vi "Dashboard Main.vi"() -> ()   [LabVIEW 2014]
uses:
  Robot/Auto/Autonomous Modes.ctl
  Robot/Main/Arms/Arm clapper state.ctl
  Robot/Main/Arms/Arm State.ctl
  Dashboard Tab.ctl
  <vilib>/event_ctls.llb/eventvkey.ctl
  <vilib>/vision/Image Controls.llb/IMAQ Image.ctl
  <vilib>/Rock Robotics/WPI/Dashboard/WPI_DashboardLogging Global.vi
  <vilib>/Rock Robotics/Network Tables/SD Write Number.vi
  <vilib>/Rock Robotics/Network Tables/SD Read Number.vi
  <vilib>/Rock Robotics/Network Tables/SD Write Boolean.vi
  <vilib>/Utility/config.llb/Write Key (String).vi
  <vilib>/Utility/config.llb/Write Key (I32).vi
  <vilib>/Utility/config.llb/NI_LVConfig.lvlib
  <vilib>/vision/NI_Vision_Development_Module.lvlib
panel:
  in  "Rec Mode":enum32{"Stop", "Record", "Playback"}(radio)
  in  "Vision":u16(ring) items=["Camera Off", "USB Camera SW", "USB Camera HW", "IP Camera"]
  out "fps":dbl format="%#.1g"
  out "Mbps":dbl format="%#.1g"
  out "Mbps 2":bool
  in  "TCP":refnum<k5>
  out "Camera IP":string
  out "Image Message":string="Timeout in Camera Communications"
  out "Camera Image":T1(plugin-control)
  in  "Dashboard Tab":T2(tab)
  out "Clapper Manual":bool caption="Clapper"
  out "Arm Angle Manual":bool caption="Arms"
  out "Elevator Manual":bool caption="Elevator"
  out "Arm Angle POT":dbl caption="Arm Angle"
  out "Clapper POT":dbl caption="Clapper"
  out "Left Drive Encoder":dbl caption="Left Drive"
  out "Right Drive Encoder":dbl caption="Right Drive"
  out "Elevator Encoder":dbl caption="Elevator"
  out "Version":string
  out "Arm Angle Ground":bool
  out "Arm Angle Level":bool
  out "Arm Angle Feeder":bool
  out "Arm Angle Vertical":bool
  out "Arm Angle":T3
  out "Clapper In":bool
  out "Clapper Tote":bool
  out "Clapper Bin":bool
  out "Clapper Out":bool
  out "Clapper":T4
  out "Clapper Straight":bool
  out "Motor Ramp":bool caption="Ramp"
  out "Half Drive":bool caption="Half"
  out "Mode":T5(ring)=enum."Auto Disabled"
  out "Elevator":u16
  out "Ground":bool
  out "Tote 1":bool
  out "Tote 2":bool
  out "Tote 3":bool
  out "Tote 4":bool
  out "Tote 5":bool
  out "Gyro Indicator":dbl(knob) scale=0.0..360.0
  out "Bottom LS":bool
  out "Top LS":bool
  out "Tote Detect":bool
  in  "Auto Modes":T6
  in  "DB Camera Config":bool
  in  "Camera Settings":T7={"Frame Rate"=30, "Compression"=30, "Size"=1} {"Frame Rate" scale=1.0..30.0; "Size" items=["640x480", "320x240", "160x120"]}
  in  "Test Slider":dbl(slide) scale=0.0..100.0 scale format="%#_3g"
  in  "On/Off":bool caption="Solenoid"
  in  "Test Name":u16(ring) items=["Select the test to run..."]
  in  "Test Tree":string(tree)
  in  "Motor":cluster{"Value":dbl, "Enable":bool} {"Value" scale=-1.0..1.0 scale format="%#_3g"}
  out "Progress":T8 {"Test Progress" scale=0.0..100.0}
  in  "Rev/Fwd":cluster{"Forward":bool, "Reverse":bool}
  in  "Test Ring":u16(ring) items=["Monochrome", "Color"]
  in  "Listbox":i32(listbox)
  out "Tree":string(tree)
  in  "Strafe Ramp":dbl(slide)=0.5 min=0.1 max=5.0 step=1e-06 scale=0.0..1.0
  in  "Rotate Sensitivity":dbl(slide)=1.0 min=0.0 max=1.0 step=0.05 scale=0.0..1.0
  in  "Strafe Sensitivity":dbl(slide)=1.0 min=0.0 max=1.0 step=0.05 scale=0.0..1.0
  in  "Motor Ramp":dbl(slide)=0.5 min=0.1 max=5.0 step=1e-06 scale=0.0..1.0
  in  "Joystick Curve Power":dbl=1.0 min=0.5 max=4.0 step=0.5
  in  "Elevator PIDs":bool
  in  "Strafe PIDs":bool
  in  "Arm PIDs":bool
  out "Boolean":bool
  # "POTENTIOMETERS"
  # "ENCODERS"
  # "Elevator LS"
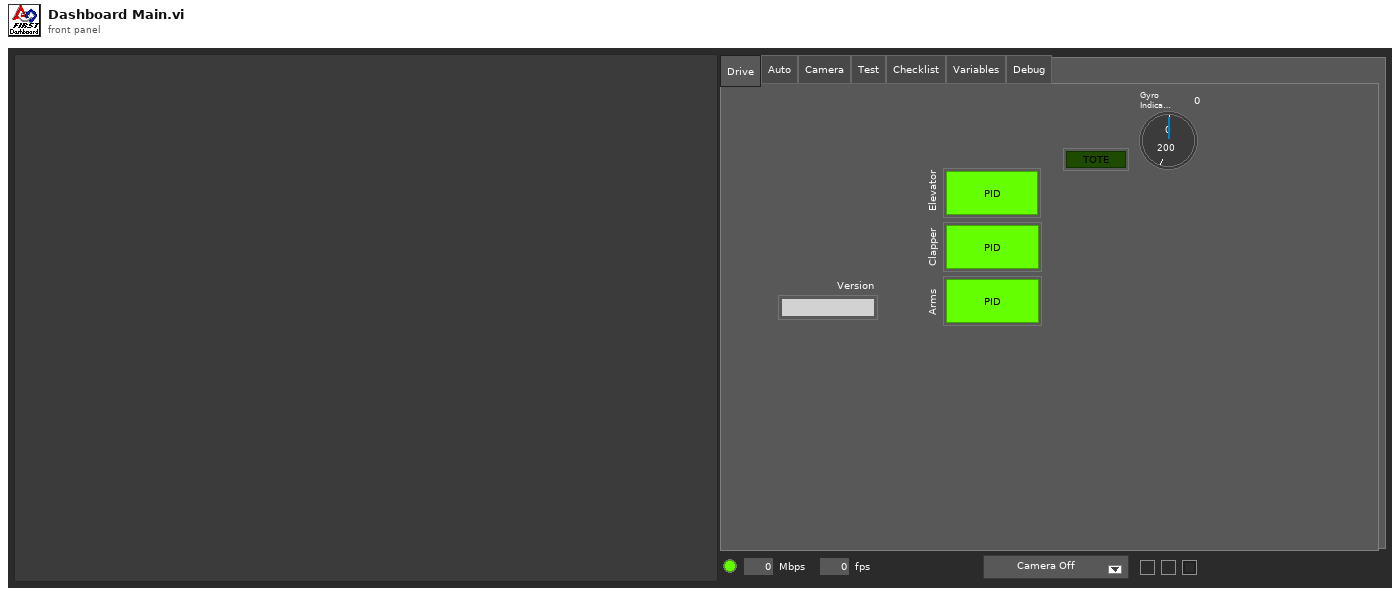
[diagram p1: front panel]
types:
  T1 = typedef "IMAQ Image.ctl" = refnum<image>
  T2 = enum32{"Drive", "Auto", "Camera", "Test", "Checklist", "Variables", "Debug"}
  T3 = typedef "Arm State.ctl" = enum16{"Ground", "Level", "Feeder", "Vertical"}
  T4 = typedef "Arm clapper state.ctl" = enum16{"In", "Tote Closed", "Bin Closed", "Straight", "Open"}
  T5 = enum8{"Tele-Op Disabled", "Tele-Op Enabled", "Auto Disabled", "Auto Enabled", "Test Disabled", "Test Enabled", "Disconnected", "No Code", "E-Stop"}
  T6 = typedef "Autonomous Modes.ctl" = enum16{"3 Tote", "Turn Left, Drive to Auto", "Turn Right, Drive to Auto", "1 Bin", "Move To Auto Zone", "Do Nothing"}
  T7 = cluster{"Frame Rate":i32, "Compression":i32, "Size":u16}
  T8 = cluster{"Test Progress":u8, "Test Progress Text":string}
  T9 = typedef "Dashboard Tab.ctl" = enum16{"Drive", "Auto", "Camera", "Test", "Checklist", "Variables", "Debug"}
  T10 = typedef "Image Type" = u32
  T11 = cluster{"Camera Image":refnum<vi>, "Dashboard Tab":refnum<vi>, "Boolean":refnum<vi>, "Vision":refnum<vi>, "Rec Mode":refnum<vi>, "Test Slider":refnum<vi>, "On/Off ":refnum<vi>, "Test Ring":refnum<vi>, "Rev/Fwd":refnum<vi>, "Test Name":refnum<vi>, "Motor":refnum<vi>, "Progress":refnum<vi>, "CheckList":refnum<vi>, "Tree":refnum<vi>, "Test Tree":refnum<vi>}
  T12 = cluster{"Error Strings":string, "Disable Counts":cluster{u16, u16}, "Rail Faults":cluster{u16, u16, u16}, "Robot IP":string, "DB Mode":u8, "Event Info":cluster{"Name":string, "Type":u8, "Number":u16, "Replay":u8}, "Camera Addr":string}
  T13 = cluster{"Storage":cluster{"Disk Free":u64, "RAM Block":u32, "RAM free":u32}, "CPU Utilization":cluster{"CPU % ISR":sgl, "CPU % Time Crit":sgl, "CPU % Timed Str":sgl, "CPU % High":sgl, "CPU % Above":sgl, "CPU % Normal":sgl, "CPU % Low":sgl}, "CAN":cluster{"% Bus Utilization":sgl, "Bus Off Cnt":u32, "TX_FIFO Full Cnt":u32, "Receive Error Cnt":u8, "Transmit Error Cnt":u8}, "HID":cluster{"HID Outputs":u32, "Rumble Low":u16, "Rumble High":u16}[]}
  T14 = cluster{"Status bits":cluster{"Test Mode":bool, "Autonomous":bool, "Enabled":bool, "Code Start":bool, "Brownout":bool, "Reserved 2":bool, "Reserved 3":bool, "E-Stop":bool}, "Code Trace":cluster{"Disabled":bool, "TeleOp":bool, "Auto":bool, "Test":bool}, "Controller Type":enum16{"unknown", "cRIO", "roboRio"}, "Code?":enum16{"unknown", "noCode", "code"}, "Battery V":dbl}
  T15 = cluster{"Control Bits":cluster{"TestMode":bool, "Autonomous":bool, "Enabled":bool, "FMS Present":bool, bool, bool, bool, "E-Stop":bool}, "Team Station ":u8, "Countdown":sgl, "Joystick Values":cluster{"Axes":dbl[], "Buttons":bool[], "POVs":i16[]}[]}
  T16 = cluster{"Axes":dbl[], "Buttons":bool[], "POVs":i16[]}[]
  T17 = cluster{"Axes":dbl[], "Buttons":bool[], "POVs":i16[]}
  T18 = typedef "NI_LVConfig.lvlib/Config Data RefNum.ctl" = refnum<k1>
  T19 = cluster{"Operation":enum16{"Update", "Clear"}, "Color Box":u32}[]
  T20 = typedef "eventvkey.ctl" = enum16{"ASCII", "Enter", "Return", "Shift", "Ctrl", "Alt", "Cmd", "Opt", "Caps", "NumLock", "Clear", "Break", "Up", "Down", "Left", "Right", "Insert", "Delete", "Home", "End", "PageUp", "PageDown", "Escape", "Help", "Pause", "ScrollLock", "F1", "F2", "F3", "F4", "F5", "F6", "F7", "F8", "F9", "F10", "F11", "F12", "F13", "F14", "F15", "F16", "F17", "F18", "F19", "F20", "F21", "F22", "F23", "F24", "Play", "VolumeUp", "VolumeDown", "Mute", "Two Byte Char"}
  T21 = cluster{"Image Size":bool, "Image Type":bool, "Pixel Value":bool, "ROI Information":bool, "Zoom Factor":bool}
  T22 = enum8{"Enabled", "Disabled", "Disabled and Grayed Out"}
  T23 = cluster{"Operation":enum16{"Update", "Clear"}, "Color Box":u32}
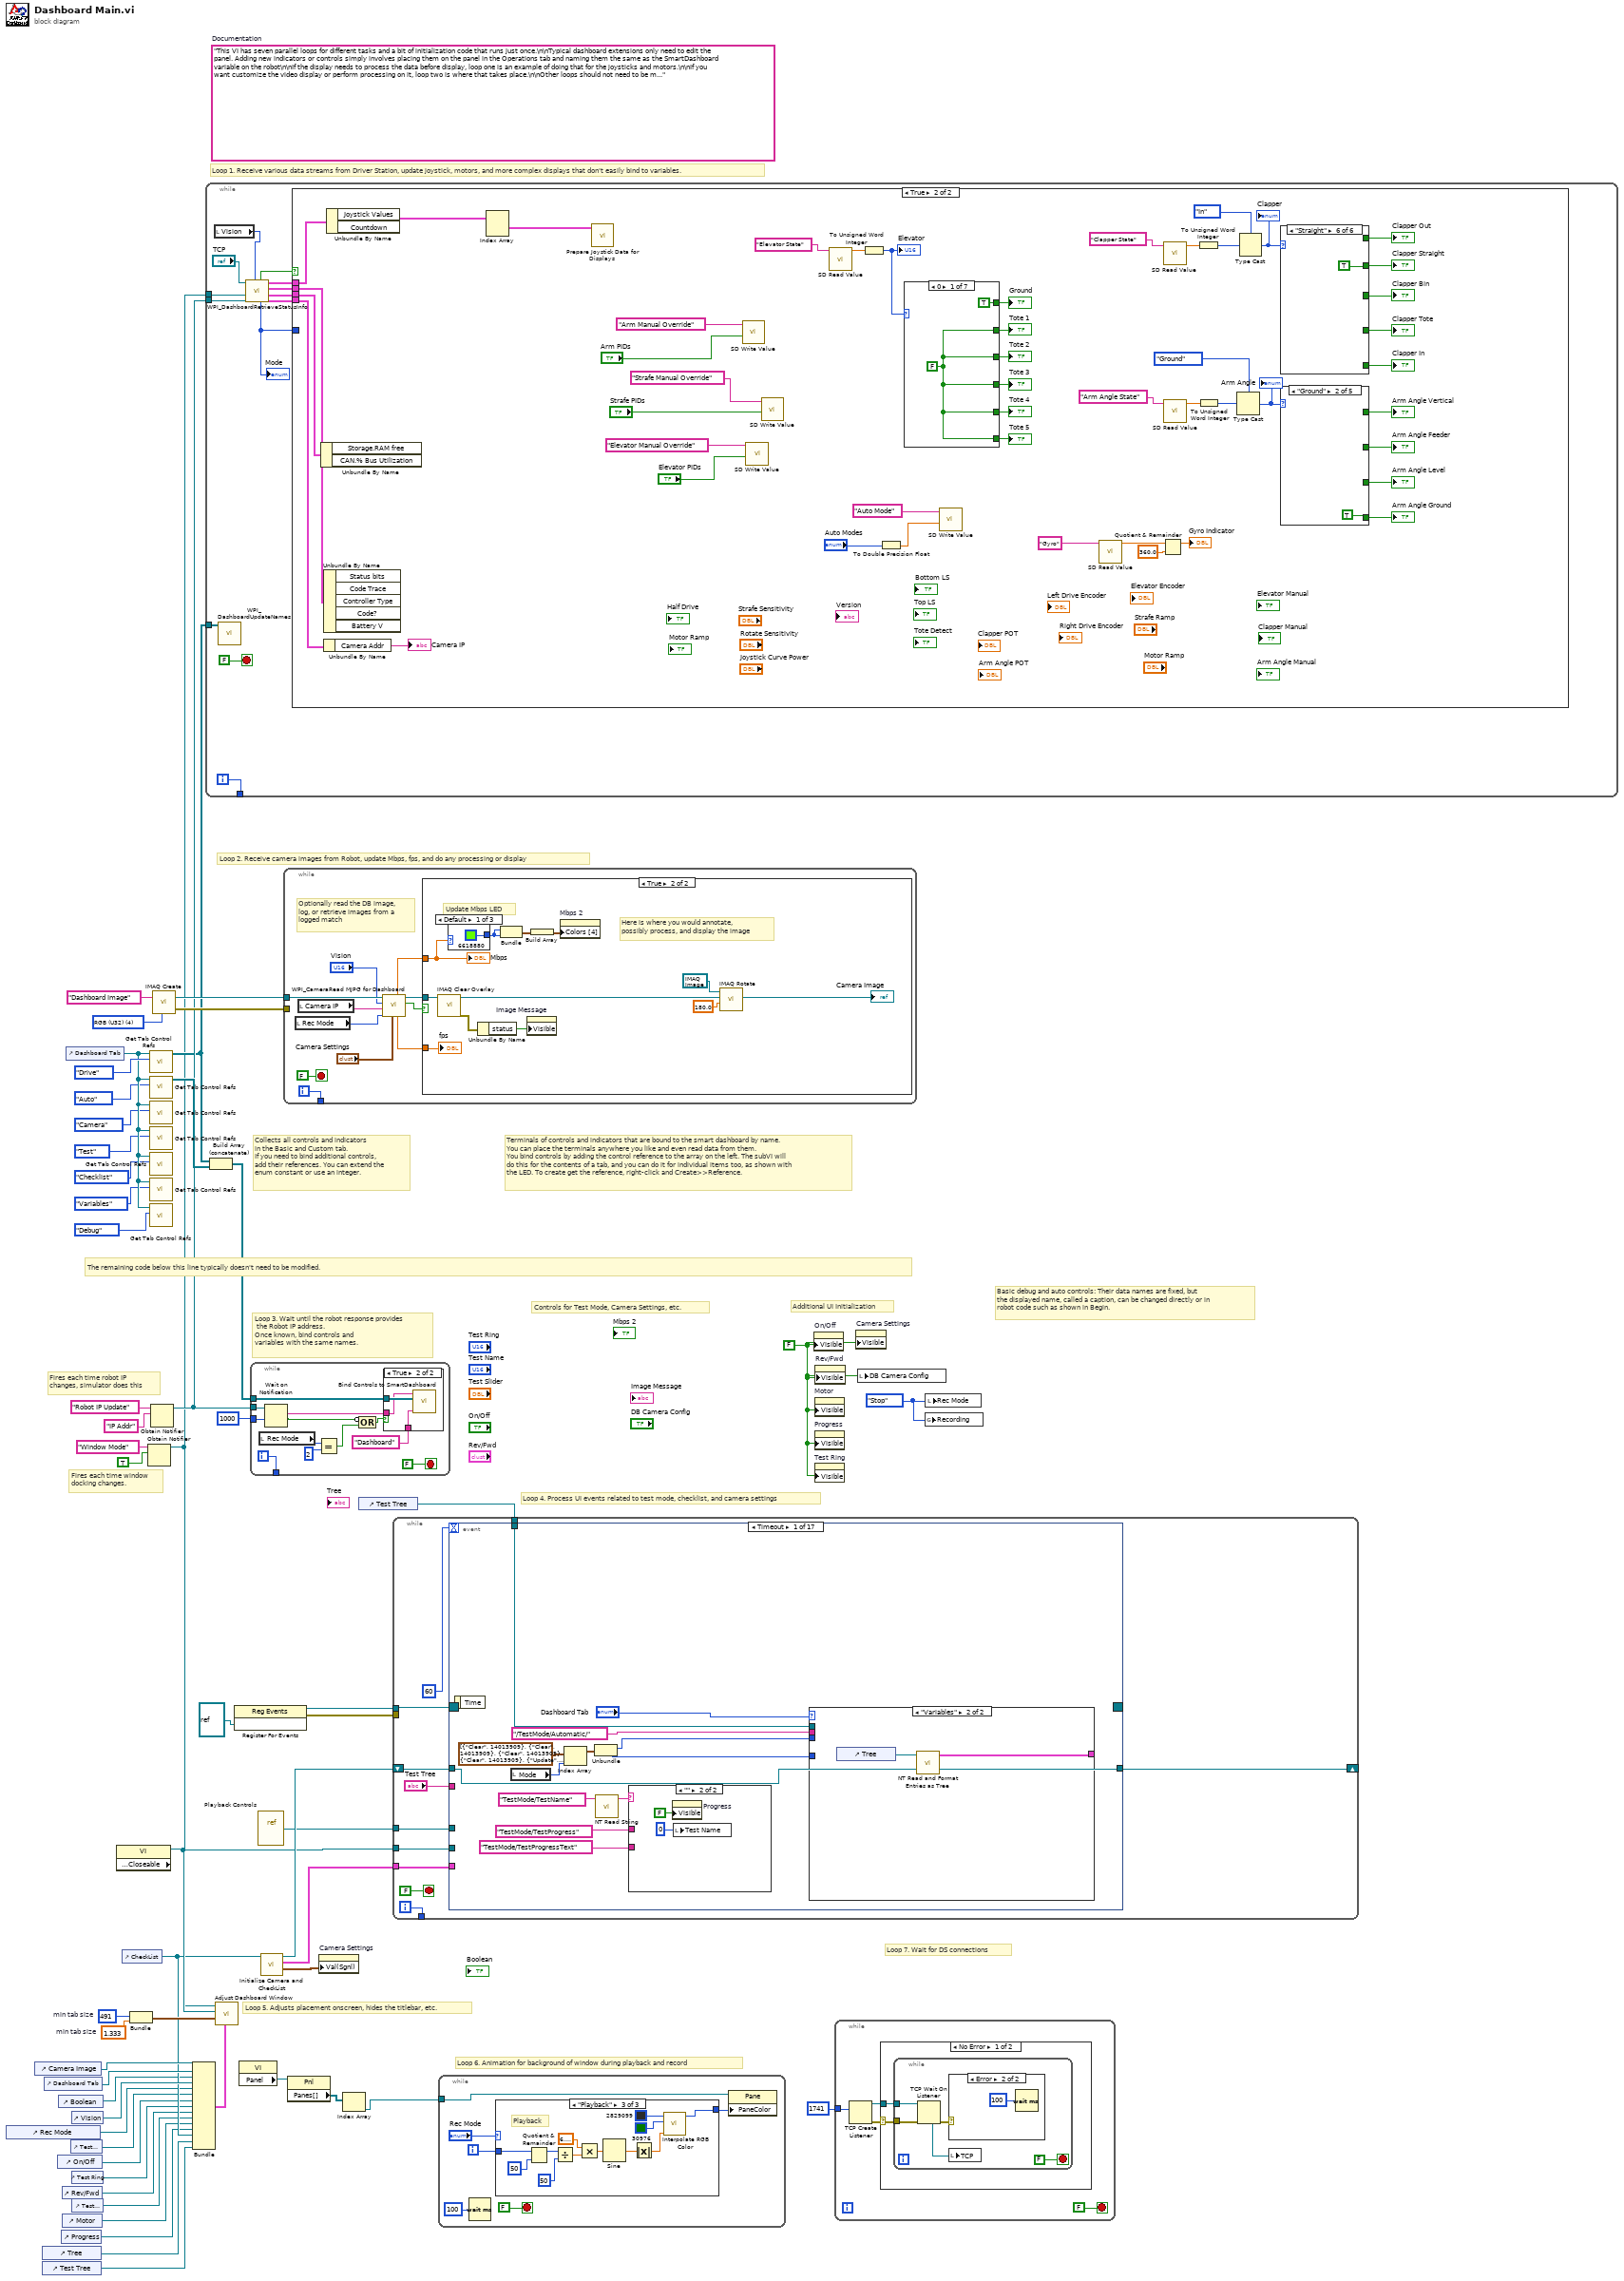
[diagram p0: block diagram]
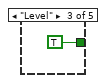
[diagram p6: hidden frame]
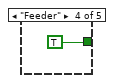
[diagram p7: hidden frame]
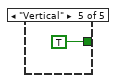
[diagram p8: hidden frame]
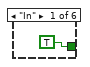
[diagram p9: hidden frame]
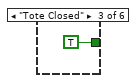
[diagram p11: hidden frame]
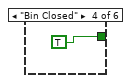
[diagram p12: hidden frame]
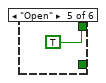
[diagram p13: hidden frame]
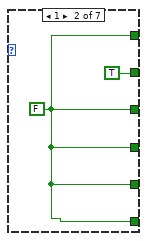
[diagram p14: hidden frame]
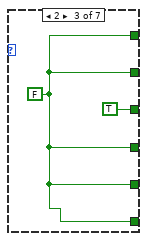
[diagram p15: hidden frame]
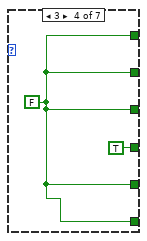
[diagram p16: hidden frame]
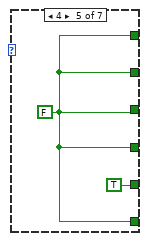
[diagram p17: hidden frame]
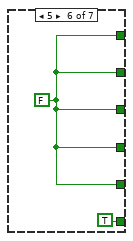
[diagram p18: hidden frame]
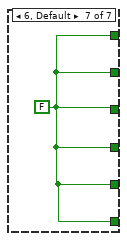
[diagram p19: hidden frame]
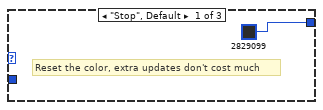
[diagram p20: hidden frame]
diagram:
  w29 = 491  # min tab size
  w28 = 1.333  # min tab size
  w36 = enum32{"Stop", "Record", "Playback"}."Stop" ("Rec Mode")
  w15 = FALSE ("Visible")
  (unwired) "This VI has seven parallel loops for different tasks and a bit of initialization code that runs just once.\n\nTypical dashboard extensions only need to edit the panel. Adding new indicators or controls simply involves placing them on the panel in the Operations tab and naming them the same as the SmartDashboard variable on the robot\n\nIf the display needs to process the data before display, loop one is an example of doing that for the joysticks and motors.\n\nIf you want customize the video display or perform processing on it, loop two is where that takes place.\n\nOther loops should not need to be modified. They are pretty standard, and document the task they perform."  # Documentation
  w56 = T10 4 items=["Grayscale (U8)", "Grayscale (I16)", "Grayscale (SGL)", "Complex (CSG)", "RGB (U32)", "HSL (U32)", "RGB (U64)"] ("Image Type")
  # "Loop 7. Wait for DS connections"
  # "Basic debug and auto controls: Their data names are fixed, but\nthe displayed name, called a caption, can be changed directly or in\nrobot code such as shown in Begin."
  # "Controls for Test Mode, Camera Settings, etc."
  # "Additional UI Initialization"
  # "Loop 6. Animation for background of window during playback and record"
  # "Fires each time robot IP\nchanges, simulator does this"
  # "Fires each time window\ndocking changes."
  # "Collects all controls and indicators\nin the Basic and Custom tab.\nIf you need to bind additional controls,\nadd their references. You can extend the\nenum constant or use an integer."
  # "The remaining code below this line typically doesn't need to be modified."
  # "Loop 4. Process UI events related to test mode, checklist, and camera settings"
  # "Terminals of controls and indicators that are bound to the smart dashboard by name.\nYou can place the terminals anywhere you like and even read data from them.\nYou bind controls by adding the control reference to the array on the left. The subVI will\ndo this for the contents of a tab, and you can do it for individual items too, as shown with\nthe LED. To create get the reference, right-click and Create>>Reference."
  # "Loop 3. Wait until the robot response provides\n the Robot IP address.\nOnce known, bind controls and\nvariables with the same names."
  # "Loop 5. Adjusts placement onscreen, hides the titlebar, etc."
  # "Loop 1. Receive various data streams from Driver Station, update joystick, motors, and more complex displays that don't easily bind to variables."
  # "Loop 2. Receive camera images from Robot, update Mbps, fps, and do any processing or display"
  n1 = control-ref of="Rec Mode"() -> (w21:refnum<vi>)
  n2 = control-ref of="Camera Image"() -> (w32:refnum<vi>)
  n3 = control-ref of="Tree"() -> (w25:refnum<vi>)
  n4 = control-ref of="Test Tree"() -> (w24:refnum<vi>)
  n5 = control-ref of="Dashboard Tab"() -> (w31:refnum<vi>)
  n6 = control-ref of="On/Off"() -> (w19:refnum<vi>)
  n7 = control-ref of="Boolean"() -> (w1:refnum<vi>)
  n8 = control-ref of="Progress"() -> (w16:refnum<vi>)
  n9 = control-ref of="Rev/Fwd"() -> (w17:refnum<vi>)
  n10 = control-ref of="Motor"() -> (w22:refnum<vi>)
  n11 = control-ref of="Dashboard Tab"() -> (w9:refnum<vi>)
  n12 = control-ref of="Test Slider"() -> (w20:refnum<vi>)
  n13 = control-ref of="Vision"() -> (w30:refnum<vi>)
  n14 = control-ref of="Test Ring"() -> (w18:refnum<vi>)
  n15 = control-ref of="Test Name"() -> (w23:refnum<vi>)
  n16 = property class="VI" props=["Front Panel.Closeable"]() -> (reference out=w35:refnum<vi>)  [unwired: 2 in, 2 out]
  n17 = control-ref of="CheckList"() -> (w26:refnum<vi>)
  n18 = Bundle("min tab size"=w29, "min tab size"=w28) -> (w27:cluster{"min tab size":i32, "min tab size":dbl})  [unwired: 1 in]
  n19 = Obtain Notifier(name (unnamed)="Window Mode", notification data type=TRUE) -> (notifier out=w12:refnum<notifier>)  [unwired: 2 in, 2 out]
  n20 = call <vilib>:"Get Tab Control Refs.vi"("Page Index"=Dashboard_Tab."Drive", "TabControl in"=w9) -> ("ControlsOnPage"=w13:refnum<vi>[])  [unwired: 9 in]
  n21 = call <vilib>:"Get Tab Control Refs.vi"("Page Index"=Dashboard_Tab."Auto", "TabControl in"=w9) -> ("ControlsOnPage"=w34:refnum<vi>[])  [unwired: 9 in]
  n22 = call <vilib>:"Get Tab Control Refs.vi"("Page Index"=Dashboard_Tab."Camera", "TabControl in"=w9) -> ()  [unwired: 9 in, 1 out]
  n23 = call <vilib>:"Get Tab Control Refs.vi"("Page Index"=Dashboard_Tab."Test", "TabControl in"=w9) -> ()  [unwired: 9 in, 1 out]
  n24 = call <vilib>:"Get Tab Control Refs.vi"("Page Index"=Dashboard_Tab."Checklist", "TabControl in"=w9) -> ()  [unwired: 9 in, 1 out]
  n25 = call <vilib>:"Get Tab Control Refs.vi"("Page Index"=Dashboard_Tab."Variables", "TabControl in"=w9) -> ()  [unwired: 9 in, 1 out]
  n26 = call <vilib>:"Get Tab Control Refs.vi"("Page Index"=Dashboard_Tab."Debug", "TabControl in"=w9) -> ()  [unwired: 9 in, 1 out]
  n27 = Obtain Notifier(name (unnamed)="Robot IP Update", notification data type="IP Addr" ("name (unnamed)")) -> (notifier out=w14:refnum<notifier>)  [unwired: 2 in, 2 out]
  n28 = call "IMAQ Create"("Image Name"="Dashboard Image", "Image Type"=w56) -> ("New Image"=w54:T1, "error out"=w53:errorcluster)  [unwired: 2 in, 1 out]
  n29 = Bundle("Camera Image"=w32, "Dashboard Tab"=w31, "Boolean"=w1, "Vision"=w30, "Rec Mode"=w21, "Test Slider"=w20, "On/Off"=w19, "Test Ring"=w18, "Rev/Fwd"=w17, "Test Name"=w23, "Motor"=w22, "Progress"=w16, "CheckList"=w26, "Tree"=w25, "Test Tree"=w24) -> (w2:T11)  [unwired: 1 in]
  n30 = while {
    tunnel: [w68] -> _
    tunnel: w14 -> [w62]
    tunnel: w13 -> [w61]
    tunnel: w12 -> [w57]
    i -> [w68]
    stop <- FALSE stop-if-true
    n31 = local read "Vision"() -> (w59:u16)
    n32 = call <vilib>:"WPI_DashboardUpdateNames.vi"("Controls on Tab"=w61) -> ()  [unwired: 11 in]
    n33 = call <vilib>:"WPI_DashboardRetrieveStatusInfo.vi"("Vision"=w59, "Binding Refnum"=w62, "Window Mode Notifier"=w57, "TCP Cnx"="TCP") -> ("Power and Errors"=w63:T12, "Robot Metrics"=w66:T13, "Status Info"=w67:T14, "Control Info"=w64:T15, "Robot Mode"=w60:T5, "Process?"=w65:bool)  [unwired: 2 in]
    "Mode" <- w60
    n34 = case shown="True" w65 {
      tunnel: w67 -> [_ w117]
      tunnel: w66 -> [_ w116]
      tunnel: w64 -> [_ w115]
      tunnel: w63 -> [_ w114]
      tunnel: w60 -> [_ _]
      frame False {
      }
      frame True {
        n35 = Unbundle By Name(w116) -> ()  [unwired: 2 out]
        n36 = Unbundle By Name(w114) -> ("Camera Addr"=→"Camera IP":string)
        n37 = Unbundle By Name(w117) -> ()  [unwired: 5 out]
        n38 = Unbundle By Name(w115) -> ("Joystick Values"=w113:T16)  [unwired: 1 out]
        n39 = Index Array(array=w113) -> (element #1=w111:T17)  [unwired: 2 in, 1 out]
        n40 = call "Prepare Joystick Data for Displays.vi"("Joystick Values"=w111) -> ()  [unwired: 8 in, 3 out]
        n41 = call-poly <vilib>:"SD Write Value.vi"("Boolean"="Arm PIDs", "Name"="Arm Manual Override") -> ()  [unwired: 8 in, 2 out]
        n42 = call-poly <vilib>:"SD Write Value.vi"("Boolean"="Elevator PIDs", "Name"="Elevator Manual Override") -> ()  [unwired: 8 in, 2 out]
        n43 = call-poly <vilib>:"SD Write Value.vi"("Boolean"="Strafe PIDs", "Name"="Strafe Manual Override") -> ()  [unwired: 8 in, 2 out]
        n44 = call-poly <vilib>:"SD Read Value.vi"("Name"="Elevator State") -> ("Numeric"=w107:dbl)  [unwired: 8 in, 2 out]
        n45 = To Unsigned Word Integer(number=w107) -> (unsigned 16bit integer=w105:u16)
        "Elevator" <- w105
        n46 = To Double Precision Float(number="Auto Modes") -> (double precision float=w109:dbl)
        n47 = case shown="0" w105 {
          tunnel: [TRUE ("Ground") w129 w131 w133 w135 w137 w139] -> w104
          tunnel: [w127 w129 w131 w133 w135 TRUE w139] -> w103
          tunnel: [w127 w129 w131 w133 TRUE w137 w139] -> w102
          tunnel: [w127 w129 w131 TRUE w135 w137 w139] -> w101
          tunnel: [w127 w129 TRUE w133 w135 w137 w139] -> w100
          tunnel: [w127 TRUE w131 w133 w135 w137 w139] -> w99
          frame 0 {
            w127 = FALSE
          }
          frame 1 {
            w129 = FALSE
          }
          frame 2 {
            w131 = FALSE
          }
          frame 3 {
            w133 = FALSE
          }
          frame 4 {
            w135 = FALSE
          }
          frame 5 {
            w137 = FALSE
          }
          frame 6, Default {
            w139 = FALSE
          }
        }
        "Ground" <- w104
        "Tote 1" <- w99
        "Tote 2" <- w100
        "Tote 3" <- w101
        "Tote 4" <- w102
        "Tote 5" <- w103
        n48 = call-poly <vilib>:"SD Write Value.vi"("Numeric"=w109, "Name"="Auto Mode") -> ()  [unwired: 8 in, 2 out]
        n49 = call-poly <vilib>:"SD Read Value.vi"("Name"="Gyro") -> ("Numeric"=w78:dbl)  [unwired: 8 in, 2 out]
        n50 = Quotient & Remainder(x=w78, y=360.0) -> (x-y*floor(x/y)=→"Gyro Indicator":dbl)  [unwired: 1 out]
        n51 = call-poly <vilib>:"SD Read Value.vi"("Name"="Clapper State") -> ("Numeric"=w98:dbl)  [unwired: 8 in, 2 out]
        n52 = call-poly <vilib>:"SD Read Value.vi"("Name"="Arm Angle State") -> ("Numeric"=w96:dbl)  [unwired: 8 in, 2 out]
        n53 = To Unsigned Word Integer(number=w98) -> (unsigned 16bit integer=w94:u16)
        n54 = To Unsigned Word Integer(number=w96) -> (unsigned 16bit integer=w91:u16)
        n55 = Type Cast(type=Arm_State."Ground" ("Enum"), x=w91) -> (*(type *) &x=w90:T3)
        "Arm Angle" <- w90
        n56 = Type Cast(type=Arm_clapper_state."In" ("Enum"), x=w94) -> (*(type *) &x=w93:T4)
        "Clapper" <- w93
        n57 = case shown="\"Straight\"" w93 {
          tunnel: [_ _ _ _ TRUE _] -> w88
          tunnel: [_ _ _ TRUE _ _] -> w87
          tunnel: [_ _ TRUE _ _ _] -> w86
          tunnel: [TRUE _ _ _ _ _] -> w85
          tunnel: [_ _ _ _ _ TRUE] -> w76
          frame "In" {
          }
          frame Default {
          }
          frame "Tote Closed" {
          }
          frame "Bin Closed" {
          }
          frame "Open" {
          }
          frame "Straight" {
          }
        }
        "Clapper Out" <- w88
        "Clapper Bin" <- w87
        "Clapper Tote" <- w86
        "Clapper In" <- w85
        "Clapper Straight" <- w76
        n58 = case shown="\"Ground\"" w90 {
          tunnel: [_ _ _ _ TRUE] -> w84
          tunnel: [_ _ _ TRUE _] -> w83
          tunnel: [_ _ TRUE _ _] -> w82
          tunnel: [_ TRUE _ _ _] -> w81
          frame Default {
          }
          frame "Ground" {
          }
          frame "Level" {
          }
          frame "Feeder" {
          }
          frame "Vertical" {
          }
        }
        "Arm Angle Vertical" <- w84
        "Arm Angle Feeder" <- w83
        "Arm Angle Level" <- w82
        "Arm Angle Ground" <- w81
      }
    }
  }
  n59 = Build Array (concatenate)(w13, w34) -> (w33:refnum<vi>[])
  n60 = call "Adjust Dashboard Window.vi"("Sizing Refnums"=w2, "Size Constraints"=w27, "VI"=w35, "Notifier in"=w12) -> ()  [unwired: 8 in]
  n61 = register-events(refnum<vi> refnum) -> (reference out=w40:refnum<event-registration>, error out=w39:errorcluster)  [unwired: 2 in]
  n62 = property class="VI"() -> ("Panel"=w43:refnum<vi>)  [unwired: 2 in, 2 out]
  n63 = while {
    tunnel: w33 -> [w151]
    tunnel: w14 -> [w149]
    tunnel: [w147] -> _
    tunnel: u32 1000 ("milliseconds to wait") -> [w146]
    i -> [w147]
    stop <- FALSE stop-if-true
    n64 = local read "Rec Mode"() -> (w142:enum32{"Stop", "Record", "Playback"})
    n65 = Wait on Notification(notifier=w149, timeout in ms (-1)=w146) -> (notification=w148:string, timed out?=w144:bool)  [unwired: 2 in, 2 out]
    n66 = Equal?(x=w142, y=u16 2 ("Rec Mode")) -> (x = y?=w143:bool)
    n67 = Compound Arithmetic op=OR(invert w144, w143) -> (w145:bool)
    n68 = case shown="True" w145 {
      tunnel: w151 -> [_ w154]
      tunnel: w148 -> [_ w153]
      tunnel: "Dashboard" -> [_ w152]
      frame False {
      }
      frame True {
        n69 = call <vilib>:"Bind Controls to SmartDashboard.vi"("Client Name"=w152, "Bound Control Refs"=w154, "Server IP Address"=w153) -> ()  [unwired: 9 in]
      }
    }
  }
  n70 = vi-ref "Playback Controls.vi"() -> (w41:refnum<vi>)
  n71 = call "Initialize Camera and CheckList.vi"("ListBox in"=w26) -> ("Cluster"=w47:cluster{"value":i32, "value":i32, "index":i32}, "Array"=w48:cluster{string[]}[], "File Refnum"=w46:T18)  [unwired: 8 in]
  n72 = while {
    tunnel: w54 -> [w163]
    tunnel: w53 -> [_]
    tunnel: [w164] -> _
    i -> [w164]
    stop <- FALSE stop-if-true
    # "Optionally read the DB image,\nlog, or retrieve images from a\nlogged match"
    n73 = local read "Rec Mode"() -> (w157:enum32{"Stop", "Record", "Playback"})
    n74 = local read "Camera IP"() -> (w155:string)
    n75 = call <vilib>:"WPI_CameraRead MJPG for Dashboard.vi"("Camera Settings"="Camera Settings", "Rec Mode"=w157, "Camera IP"=w155, "Camera Mode"="Vision", "Refnum in"=w163) -> ("Active"=w161:bool, "Refnum out"=w162:T1, "FPS"=w160:dbl, "Bandwidth (Mbps)"=w159:dbl)  [unwired: 3 in]
    n76 = case shown="True" w161 {
      tunnel: w162 -> [_ w173]
      tunnel: w159 -> [_ w172]
      tunnel: w160 -> [_ w170]
      frame False {
        # "Sleep for 500ms"
        n77 = Wait Until Next ms Multiple(millisecond multiple=u32 500) -> ()  [unwired: 1 out]
      }
      frame True {
        # "Here is where you would annotate,\npossibly process, and display the image"
        # "Update Mbps LED"
        n78 = call "IMAQ Clear Overlay"("Image"=w173) -> ("error out"=w177:errorcluster, "Image Out"=w171:T1)  [unwired: 2 in, 7 out]
        n79 = case shown="Default" w172 {
          tunnel: [u32 6618880 ("Color Box") u32 16776722 ("Color Box") u32 16716800 ("Color Box")] -> w174
          frame Default {
          }
          frame 4, 5 {
          }
          frame 6.. {
          }
        }
        n80 = Unbundle By Name(w177) -> ("status"=w178:bool)
        n81 = Bundle("Color Box"=w174, "Color Box"=w174) -> (w176:cluster{"Color Box":u32, "Color Box":u32})  [unwired: 1 out]
        n82 = property on="Image Message" class="Str"("Visible"=w178) -> ()  [unwired: 2 in, 2 out]
        n83 = Build Array(w176) -> (w175:cluster{"Color Box":u32, "Color Box":u32}[])
        n84 = property on="Mbps 2" class="Bool (strict)"("Colors [4]"=w175) -> ()  [unwired: 2 in, 2 out]
        n85 = call "IMAQ Rotate"("Angle (degrees)"=sgl 180.0, "Image Dst"=w171, "Image Src"=T1 refnum) -> ("Image Dst Out"=→"Camera Image":T1)  [unwired: 7 in, 1 out]
        "Mbps" <- w172
        "fps" <- w170
      }
    }
  }
  n86 = property class="Pnl"(reference=w43) -> ("Panes[]"=w44:refnum<vi>[])  [unwired: 1 in, 2 out]
  n87 = property on="Camera Settings" class="Clust (strict)"("Val(Sgnl)"=w47) -> ()  [unwired: 2 in, 2 out]
  n88 = Index Array(array=w44) -> (element=w42:refnum<vi>)  [unwired: 1 in]
  n89 = control-ref of="Test Tree"() -> (w45:refnum<vi>)
  n90 = while {
    tunnel: w48 -> [w189]
    shift-right: [w188] -> _
    shift-left: w46 -> [w187]
    tunnel: [w186] -> _
    tunnel: w45 -> [w185]
    tunnel: w41 -> [w184]
    tunnel: w40 -> [w183]
    tunnel: w39 -> [_]
    tunnel: w35 -> [w182]
    i -> [w186]
    stop <- FALSE stop-if-true
    n91 = event shown="[0] Timeout" {
      selector: w183 -> [_ _ _ _ _ _ _ _ _ _ _ _ _ _ _ _ _]
      dyn-events: [_ _ _ _ _ _ _ _ _ _ _ _ _ w427 _ _ _] -> _
      timeout: u32 60 ("milliseconds to wait") -> [_ _ _ _ _ _ _ _ _ _ _ _ _ _ _ _ _]
      tunnel: w185 -> [w201 _ _ _ _ _ _ _ _ _ _ _ _ _ _ _ _]
      tunnel: "Test Tree" -> [_ _ _ _ _ _ _ _ w396 w404 w406 w410 w418 _ _ _ _]
      tunnel: w189 -> [_ w223 _ _ _ _ w360 w390 _ _ _ _ _ _ _ _ _]
      tunnel: [w197 w222 w321 w326 w334 w346 w359 w383 w395 w402 w405 w409 w417 w429 w443 w444 w454] -> w188
      tunnel: w187 -> [w197 w222 w321 w326 w334 w346 w358 w383 w395 w402 w405 w409 w417 w429 w443 w444 w454]
      tunnel: w184 -> [_ _ _ _ _ _ _ _ _ _ _ _ _ w430 _ w447 _]
      tunnel: w182 -> [_ _ _ _ _ _ _ _ _ _ _ _ _ w425 _ _ _]
      event Timeout {
        n92 = event-data() -> ()  [unwired: 1 in, 1 out]
        n93 = local read "Mode"() -> (w200:T5)
        n94 = Index Array(array=T19 [{"Operation"=enum."Clear", "Color Box"=14013909}, {"Operation"=enum."Clear", "Color Box"=14013909}, {"Operation"=enum."Clear", "Color Box"=14013909}, {"Operation"=enum."Clear", "Color Box"=14013909}, {"Operation"=enum."Update", "Color Box"=14013909}, {"Operation"=enum."Update", "Color Box"=16777215}, {"Operation"=enum."Clear", "Color Box"=14013909}, {"Operation"=enum."Clear", "Color Box"=14013909}, {"Operation"=enum."Clear", "Color Box"=14013909}], index=w200) -> (element=w195:T23)
        n95 = Unbundle(w195) -> ("Operation"=w194:enum16{"Update", "Clear"}, "Color Box"=w193:u32)
        n96 = call <vilib>:"NT Read String.vi"("Name"="TestMode/TestName") -> ("String"=w204:string)  [unwired: 9 in, 1 out]
        n97 = case shown="\"\"" w204 {
          tunnel: "TestMode/TestProgress" ("Name") -> [w216 _]
          tunnel: "TestMode/TestProgressText" ("Name") -> [w215 _]
          frame Default {
            n98 = call <vilib>:"NT Read Number.vi"("Name"=w216) -> ("Numeric"=w217:dbl)  [unwired: 9 in, 1 out]
            n99 = call <vilib>:"NT Read String.vi"("Name"=w215) -> ("String"=w218:string)  [unwired: 9 in, 1 out]
            n100 = Bundle("Numeric"=w217, "String"=w218) -> (→"Progress":cluster{"Numeric":dbl, "String":string})  [unwired: 1 in]
          }
          frame "" {
            n101 = property on="Progress" class="Clust (strict)"("Visible"=FALSE) -> ()  [unwired: 2 in, 2 out]
            n102 = local write "Test Name"(u16 0) -> ()
          }
        }
        n103 = case shown="\"Variables\"" "Dashboard Tab" {
          tunnel: w201 -> [w212 _]
          tunnel: "/TestMode/Automatic/" ("Name Pattern") -> [w211 _]
          tunnel: w194 -> [w210 _]
          tunnel: [_ w214] -> _
          tunnel: w193 -> [w206 _]
          frame "Test", Default {
            w209 = -2 ("Active Item:Row Number")
            n104 = call <vilib>:"NT Read and Format Entries as Tree.vi"("Operation"=w210, "Name Pattern"=w211, "Tree Refnum"=w212) -> ()  [unwired: 7 in, 2 out]
            n105 = property on="Test Tree" class="Tree (strict)"("Active Item Row Number"=w209, "ActiveColNum"=w209, "CellBG"=w206, "Active Item Row Number"=-1 ("Active Item:Row Number"), "CellBG"=u32 5789784 ("Color Box")) -> ()  [unwired: 2 in, 2 out]
          }
          frame "Variables" {
            n106 = control-ref of="Tree"() -> (w213:refnum<vi>)
            n107 = call <vilib>:"NT Read and Format Entries as Tree.vi"("Tree Refnum"=w213) -> ("Formatted Strings"=w214:cluster{"Name":string, "Value":string}[])  [unwired: 9 in, 1 out]
          }
        }
      }
      event "Test Tree": Value Change {
        # "Show appropriate\ncontrols"
        n108 = event-data() -> ("CtlRef"=w226:refnum<vi>, "NewVal"=w224:string)  [unwired: 1 in]
        n109 = call <vilib>:"WPI_UtilitiesGetTreeIOName.vi"("NewVal"=w224, "TreeControl in"=w226) -> ("I/O Name"=w227:string)  [unwired: 9 in]
        n110 = case shown="\"Camera\"" w227 {
          selector: w227 -> [_ w234 _ w252 w261 _]
          tunnel: w224 -> [_ _ w249 w251 _ w268]
          tunnel: w223 -> [_ _ _ _ _ w267]
          frame Default {
            w229 = FALSE ("Visible")
            w228 = FALSE ("Visible")
            n111 = property on="Motor" class="Clust (strict)"("Visible"=w228) -> ()  [unwired: 2 in, 2 out]
            n112 = property on="Test Ring" class="Ring (strict)"("Visible"=w228) -> ()  [unwired: 2 in, 2 out]
            n113 = property on="Rev/Fwd" class="Clust (strict)"("Visible"=w229) -> ()  [unwired: 2 in, 2 out]
            n114 = property on="On/Off" class="Bool (strict)"("Visible"=w229) -> ()  [unwired: 2 in, 2 out]
            n115 = property on="Test Slider" class="Slide (strict)"("Visible"=w229) -> ()  [unwired: 2 in, 2 out]
          }
          frame "Motor", "PWM" {
            w235 = FALSE ("Visible")
            n116 = case shown="\"Motor\", Default" w234 {
              tunnel: [1.0 ("Value") -1.0 ("Value")] -> w233
              tunnel: [255.0 ("Value") 1.0 ("Value")] -> w232
              tunnel: [128.0 ("Value") 0.0 ("Value")] -> w231
              tunnel: [64.0 ("Value") 0.5 ("Value")] -> w230
              frame "PWM" {
              }
              frame "Motor", Default {
              }
            }
            n117 = property on="Motor" class="Clust (strict)"("Visible"=TRUE) -> ()  [unwired: 2 in, 2 out]
            n118 = property on="Value" class="Slide (strict)"("Value"=w231, "Scale.Minimum"=w233, "Scale.Maximum"=w232, "Scale.Increment"=w230) -> ()  [unwired: 2 in, 2 out]
            n119 = property on="On/Off" class="Bool (strict)"("Visible"=w235) -> ()  [unwired: 2 in, 2 out]
            n120 = property on="Test Slider" class="Slide (strict)"("Visible"=w235) -> ()  [unwired: 2 in, 2 out]
            n121 = property on="Test Ring" class="Ring (strict)"("Visible"=w235) -> ()  [unwired: 2 in, 2 out]
            n122 = property on="Rev/Fwd" class="Clust (strict)"("Visible"=w235) -> ()  [unwired: 2 in, 2 out]
          }
          frame "Servo" {
            w247 = FALSE ("Visible")
            n123 = call <vilib>:"NT Read Number.vi"("Name"=w249) -> ("Numeric"=w248:dbl)  [unwired: 9 in, 1 out]
            n124 = property on="Test Slider" class="Slide (strict)"("Visible"=TRUE, "Scale.Maximum"=170.0 ("Scale.Range:Maximum")) -> ()  [unwired: 2 in, 2 out]
            n125 = local write "Test Slider"(w248) -> ()
            n126 = property on="Motor" class="Clust (strict)"("Visible"=w247) -> ()  [unwired: 2 in, 2 out]
            n127 = property on="Rev/Fwd" class="Clust (strict)"("Visible"=w247) -> ()  [unwired: 2 in, 2 out]
            n128 = property on="On/Off" class="Bool (strict)"("Visible"=w247) -> ()  [unwired: 2 in, 2 out]
            n129 = property on="Test Ring" class="Ring (strict)"("Visible"=w247) -> ()  [unwired: 2 in, 2 out]
          }
          frame "Relay", "Solenoid" {
            w250 = FALSE ("Visible")
            n130 = property on="Motor" class="Clust (strict)"("Visible"=w250) -> ()  [unwired: 2 in, 2 out]
            n131 = property on="Test Slider" class="Slide (strict)"("Visible"=w250) -> ()  [unwired: 2 in, 2 out]
            n132 = Search and Replace String(input string=w251, search string="/Value  **", replace string="/Direction") -> (result string=w257:string)  [unwired: 5 in, 3 out]
            n133 = property on="Test Ring" class="Ring (strict)"("Visible"=w250) -> ()  [unwired: 2 in, 2 out]
            n134 = call <vilib>:"NT Read String.vi"("Name"=w257) -> ("String"=w255:string)  [unwired: 9 in, 1 out]
            n135 = Equal?(x="Both directions", y=w255) -> (x = y?=w253:bool)
            n136 = Not(x=w253) -> (.not. x?=w254:bool)
            n137 = property on="Rev/Fwd" class="Clust (strict)"("Visible"=w253) -> ()  [unwired: 2 in, 2 out]
            n138 = property on="On/Off" class="Bool (strict)"("Visible"=w254, "Caption.Text"=w252) -> ()  [unwired: 2 in, 2 out]
          }
          frame "Compressor", "Digital Out" {
            w260 = FALSE ("Visible")
            # "Get direction and finish"
            n139 = property on="Motor" class="Clust (strict)"("Visible"=w260) -> ()  [unwired: 2 in, 2 out]
            n140 = property on="Test Slider" class="Slide (strict)"("Visible"=w260) -> ()  [unwired: 2 in, 2 out]
            n141 = property on="Test Ring" class="Ring (strict)"("Visible"=w260) -> ()  [unwired: 2 in, 2 out]
            n142 = property on="On/Off" class="Bool (strict)"("Visible"=TRUE, "Caption.Text"=w261) -> ()  [unwired: 2 in, 2 out]
            n143 = property on="Rev/Fwd" class="Clust (strict)"("Visible"=FALSE) -> ()  [unwired: 2 in, 2 out]
          }
          frame "Camera" {
            n144 = call <vilib>:"Get Last Path Segment.vi"("String in"=w268) -> ("String out"=w269:string)  [unwired: 10 in]
            n145 = property on="On/Off" class="Bool (strict)"("Visible"=FALSE) -> ()  [unwired: 2 in, 2 out]
            n146 = property on="Motor" class="Clust (strict)"("Visible"=FALSE) -> ()  [unwired: 2 in, 2 out]
            n147 = property on="Rev/Fwd" class="Clust (strict)"("Visible"=FALSE) -> ()  [unwired: 2 in, 2 out]
            n148 = case shown="\"White Balance  **\"" w269 {
              tunnel: w268 -> [w275 w284 w293 w302 w311 _ w317]
              tunnel: w267 -> [w273 w281 w290 w299 w308 _ _]
              frame "Size  **" {
                n149 = Index Array(array=w273) -> (element=w272:cluster{string[]})  [unwired: 1 in]
                n150 = call <vilib>:"NT Read String.vi"("Name"=w275) -> ("String"=w274:string)  [unwired: 9 in, 1 out]
                n151 = Unbundle(w272) -> (w270:string[])
                n152 = Match First String(2:w270, 3:w274) -> (0:w271:i32)  [unwired: 1 out]
                n153 = property on="Test Ring" class="Ring (strict)"("Value"=w271, "Strings []"=w270) -> ()  [unwired: 2 in, 2 out]
                n154 = property on="Test Ring" class="Ring (strict)"("Visible"=TRUE) -> ()  [unwired: 2 in, 2 out]
                n155 = property on="Test Slider" class="Slide (strict)"("Visible"=FALSE) -> ()  [unwired: 2 in, 2 out]
              }
              frame "White Balance  **" {
                n156 = Index Array(array=w281, index=1) -> (element=w282:cluster{string[]})
                n157 = call <vilib>:"NT Read String.vi"("Name"=w284) -> ("String"=w283:string)  [unwired: 9 in, 1 out]
                n158 = Unbundle(w282) -> (w279:string[])
                n159 = Match First String(2:w279, 3:w283) -> (0:w278:i32)  [unwired: 1 out]
                n160 = property on="Test Ring" class="Ring (strict)"("Value"=w278, "Strings []"=w279) -> ()  [unwired: 2 in, 2 out]
                n161 = property on="Test Ring" class="Ring (strict)"("Visible"=TRUE) -> ()  [unwired: 2 in, 2 out]
                n162 = property on="Test Slider" class="Slide (strict)"("Visible"=FALSE) -> ()  [unwired: 2 in, 2 out]
              }
              frame "Exposure  **" {
                n163 = Index Array(array=w290, index=2) -> (element=w291:cluster{string[]})
                n164 = call <vilib>:"NT Read String.vi"("Name"=w293) -> ("String"=w292:string)  [unwired: 9 in, 1 out]
                n165 = Unbundle(w291) -> (w287:string[])
                n166 = Match First String(2:w287, 3:w292) -> (0:w288:i32)  [unwired: 1 out]
                n167 = property on="Test Ring" class="Ring (strict)"("Value"=w288, "Strings []"=w287) -> ()  [unwired: 2 in, 2 out]
                n168 = property on="Test Ring" class="Ring (strict)"("Visible"=TRUE) -> ()  [unwired: 2 in, 2 out]
                n169 = property on="Test Slider" class="Slide (strict)"("Visible"=FALSE) -> ()  [unwired: 2 in, 2 out]
              }
              frame "Exposure Priority  **" {
                n170 = Index Array(array=w299, index=3) -> (element=w300:cluster{string[]})
                n171 = call <vilib>:"NT Read String.vi"("Name"=w302) -> ("String"=w301:string)  [unwired: 9 in, 1 out]
                n172 = Unbundle(w300) -> (w296:string[])
                n173 = Match First String(2:w296, 3:w301) -> (0:w297:i32)  [unwired: 1 out]
                n174 = property on="Test Ring" class="Ring (strict)"("Value"=w297, "Strings []"=w296) -> ()  [unwired: 2 in, 2 out]
                n175 = property on="Test Ring" class="Ring (strict)"("Visible"=TRUE) -> ()  [unwired: 2 in, 2 out]
                n176 = property on="Test Slider" class="Slide (strict)"("Visible"=FALSE) -> ()  [unwired: 2 in, 2 out]
              }
              frame "Color Enable  **" {
                n177 = Index Array(array=w308, index=4) -> (element=w309:cluster{string[]})
                n178 = call <vilib>:"NT Read String.vi"("Name"=w311) -> ("String"=w310:string)  [unwired: 9 in, 1 out]
                n179 = Unbundle(w309) -> (w305:string[])
                n180 = Match First String(2:w305, 3:w310) -> (0:w306:i32)  [unwired: 1 out]
                n181 = property on="Test Ring" class="Ring (strict)"("Value"=w306, "Strings []"=w305) -> ()  [unwired: 2 in, 2 out]
                n182 = property on="Test Ring" class="Ring (strict)"("Visible"=TRUE) -> ()  [unwired: 2 in, 2 out]
                n183 = property on="Test Slider" class="Slide (strict)"("Visible"=FALSE) -> ()  [unwired: 2 in, 2 out]
              }
              frame Default {
                n184 = property on="Test Ring" class="Ring (strict)"("Visible"=FALSE) -> ()  [unwired: 2 in, 2 out]
                n185 = property on="Test Slider" class="Slide (strict)"("Visible"=FALSE) -> ()  [unwired: 2 in, 2 out]
              }
              frame "Brightness  **", "Color Level  **", "Compression  **", "FPS  **", "Sharpness  **" {
                n186 = call <vilib>:"NT Read Number.vi"("Name"=w317) -> ("Numeric"=w316:dbl)  [unwired: 9 in, 1 out]
                n187 = local write "Test Slider"(w316) -> ()
                n188 = property on="Test Slider" class="Slide (strict)"("Visible"=TRUE, "Scale.Maximum"=100.0 ("Scale.Range:Maximum")) -> ()  [unwired: 2 in, 2 out]
                n189 = property on="Test Ring" class="Ring (strict)"("Visible"=FALSE) -> ()  [unwired: 2 in, 2 out]
              }
            }
          }
        }
        n190 = property on="Progress" class="Clust (strict)"("Visible"=FALSE) -> ()  [unwired: 2 in, 2 out]
      }
      event "Test Name": Mouse Enter {
        # "Populate the ring with the list of tests"
        n191 = event-data() -> ()  [unwired: 1 in, 1 out]
        n192 = call <vilib>:"NT Read String Array.vi"("Name"="TestMode/TestList") -> ("String Array"=w325:string[])  [unwired: 9 in, 1 out]
        n193 = Build Array (concatenate)("Select the test to run...", w325) -> (w324:string[])
        n194 = property on="Test Name" class="Ring (strict)"("Strings []"=w324) -> ()  [unwired: 2 in, 2 out]
      }
      event "Test Name": Value Change {
        w327 = FALSE ("Visible")
        # "Tell the robot the test name to run"
        n195 = event-data() -> ("NewVal"=w331:u16)  [unwired: 1 in]
        n196 = property on="Test Name" class="Ring (strict)"() -> ("Strings []"=w332:string[])  [unwired: 2 in, 2 out]
        n197 = local write "Progress"(T8 {"Test Progress"=0, "Test Progress Text"=""} ("Progress")) -> ()
        n198 = Index Array(array=w332, index=w331) -> (element=w330:string)
        n199 = call <vilib>:"NT Write String.vi"("String"=w330, "Name"="TestMode/TestName") -> ()  [unwired: 9 in, 1 out]
        n200 = property on="Progress" class="Clust (strict)"("Visible"=TRUE) -> ()  [unwired: 2 in, 2 out]
        n201 = property on="Motor" class="Clust (strict)"("Visible"=w327) -> ()  [unwired: 2 in, 2 out]
        n202 = property on="Test Slider" class="Slide (strict)"("Visible"=w327) -> ()  [unwired: 2 in, 2 out]
        n203 = property on="On/Off" class="Bool (strict)"("Visible"=w327) -> ()  [unwired: 2 in, 2 out]
        n204 = property on="Rev/Fwd" class="Clust (strict)"("Visible"=w327) -> ()  [unwired: 2 in, 2 out]
        n205 = property on="Test Ring" class="Ring (strict)"("Visible"=w327) -> ()  [unwired: 2 in, 2 out]
      }
      event "Listbox": Double Click {
        # "Shift clears all"
        # "Update symbols on the listbox"
        n206 = event-data() -> ("PlatMods.Shift"=w335:bool, "Row"=w337:i32)  [unwired: 1 in]
        n207 = case shown="True" w335 {
          tunnel: w337 -> [w341 _]
          tunnel: 1 -> [w340 _]
          frame False {
            n208 = property on="Listbox" class="LstBox (strict)"() -> ("Item Symbols"=w339:i32[])  [unwired: 2 in, 2 out]
            n209 = Replace Array Subset(array=w339, new element=w340, index=w341) -> (w338:i32[])
            n210 = property on="Listbox" class="LstBox (strict)"("Item Symbols"=w338) -> ()  [unwired: 2 in, 2 out]
          }
          frame True {
            w342 = 0 ("Top Row")
            n211 = property on="Listbox" class="LstBox (strict)"() -> ("Number of Rows"=w344:u32)  [unwired: 2 in, 2 out]
            n212 = Initialize Array(0, w344) -> (w343:i32[])
            n213 = property on="Listbox" class="LstBox (strict)"("Top Row"=w342, "Value"=w342, "Item Symbols"=w343) -> ()  [unwired: 2 in, 2 out]
          }
        }
      }
      event "Listbox": Key Down {
        # "Update symbols on the listbox\nLeft and right keys check and uncheck"
        n214 = event-data() -> ("VKey"=w348:T20)  [unwired: 1 in]
        n215 = case shown="\"Left\", \"Right\"" w348 {
          selector: w348 -> [w353 _]
          tunnel: eventvkey."Left" ("VKey") -> [w351 _]
          frame "Left", "Right" {
            n216 = Equal?(x=w351, y=w353) -> (x = y?=w352:bool)
            n217 = Select(t=0, s=w352, f=1) -> (s? t:f=w354:i32)
            n218 = property on="Listbox" class="LstBox (strict)"() -> ("Item Symbols"=w357:i32[])  [unwired: 2 in, 2 out]
            n219 = Replace Array Subset(array=w357, new element=w354, index="Listbox") -> (w356:i32[])
            n220 = property on="Listbox" class="LstBox (strict)"("Item Symbols"=w356) -> ()  [unwired: 2 in, 2 out]
          }
          frame Default {
          }
        }
      }
      event "DB Camera Config": Value Change {
        # "Show or hide the cluster of controls, store in ini file"
        n221 = event-data() -> ("NewVal"=w361:bool)  [unwired: 1 in]
        n222 = case shown="False" w361 {
          tunnel: w360 -> [w370 _]
          tunnel: [w363 w381] -> w359
          tunnel: w358 -> [w362 w381]
          frame False {
            w377 = "Camera"
            w380 = FALSE ("Visible")
            n223 = local read "Camera Settings"() -> (w369:T7)
            n224 = Index Array(array=w370) -> (element=w373:cluster{string[]})  [unwired: 1 in]
            n225 = Unbundle(w369) -> ("Frame Rate"=w368:i32, "Compression"=w367:i32, "Size"=w371:u16)
            n226 = Unbundle(w373) -> (w372:string[])
            n227 = Index Array(array=w372, index=w371) -> (element=w366:string)
            n228 = call-poly <vilib>:"Write Key.vi"("section"=w377, "value"=w366, "key"="Size", "refnum"=w362) -> ("refnum out"=w379:T18)  [unwired: 2 in, 5 out]
            n229 = call-poly <vilib>:"Write Key.vi"("section"=w377, "value"=w368, "key"="FrameRate", "refnum"=w379) -> ("refnum out"=w378:T18)  [unwired: 1 in, 6 out]
            n230 = property on="Camera Settings" class="Clust (strict)"("Visible"=w380) -> ()  [unwired: 2 in, 2 out]
            n231 = local write "DB Camera Config"(w380) -> ()
            n232 = call-poly <vilib>:"Write Key.vi"("section"=w377, "value"=w367, "key"="Compression", "refnum"=w378) -> ("refnum out"=w364:T18)  [unwired: 1 in, 6 out]
            n233 = call <vilib>:"Close Config Data.vi"("refnum"=w364) -> ("file path"=w365:path)  [unwired: 2 in, 8 out]
            n234 = call <vilib>:"Open Config Data.vi"("configuration file path"=w365) -> ("refnum"=w363:T18)  [unwired: 8 in, 2 out]
          }
          frame True {
            n235 = property on="Camera Settings" class="Clust (strict)"("Visible"=TRUE) -> ()  [unwired: 2 in, 2 out]
          }
        }
      }
      event "Camera Settings": Value Change {
        # "Update summary string when any elements of DB camera change"
        n236 = event-data() -> ("NewVal"=w394:T7)  [unwired: 1 in]
        n237 = Index Array(array=w390) -> (element=w389:cluster{string[]})  [unwired: 1 in]
        n238 = Unbundle(w394) -> ("Frame Rate"=w385:i32, "Compression"=w384:i32, "Size"=w387:u16)
        n239 = Unbundle(w389) -> (w388:string[])
        n240 = Index Array(array=w388, index=w387) -> (element=w386:string)
        n241 = Format Into String(format string="%s   %dfps   %d%%", w386, w385, w384) -> (resulting string=w391:string)  [unwired: 2 in, 1 out]
        n242 = Build Array(w391) -> (w392:string[])
        n243 = property on="DB Camera Config" class="Bool (strict)"("Strings [4]"=w392) -> ()  [unwired: 2 in, 2 out]
      }
      event "Motor.Enable": Value Change {
        # "When the test mode otor enable helper is set, update that\ntree row item's value"
        n244 = event-data() -> ("NewVal"=w400:bool)  [unwired: 1 in]
        n245 = Unbundle("Motor") -> ("Value"=w399:dbl)  [unwired: 1 out]
        n246 = Select(t=w399, s=w400, f=0.0) -> (s? t:f=w397:dbl)
        n247 = call <vilib>:"NT Write Number.vi"("Numeric"=w397, "Name"=w396) -> ()  [unwired: 9 in, 1 out]
      }
      event "Test Slider": Value Change {
        # "When the test mode slider helper is set, update that\ntree row item's value"
        n248 = event-data() -> ("NewVal"=w403:dbl)  [unwired: 1 in]
        n249 = call <vilib>:"NT Write Number.vi"("Numeric"=w403, "Name"=w404) -> ()  [unwired: 9 in, 1 out]
      }
      event "On/Off": Value Change {
        # "When the test mode on/off helper value is set, update that\ntree row item's value"
        n250 = event-data() -> ("NewVal"=w408:bool)  [unwired: 1 in]
        n251 = Boolean To (0,1)(Boolean=w408) -> (0, 1=w407:i16)
        n252 = call <vilib>:"NT Write Number.vi"("Numeric"=w407, "Name"=w406) -> ()  [unwired: 9 in, 1 out]
      }
      event "Rev/Fwd": Value Change {
        # "When the test mode helper value for relays is set, update that\ntree row item's value"
        n253 = event-data() -> ("NewVal.Forward"=w416:bool, "NewVal.Reverse"=w415:bool)  [unwired: 1 in]
        n254 = Boolean To (0,1)(Boolean=w416) -> (0, 1=w412:i16)
        n255 = Boolean To (0,1)(Boolean=w415) -> (0, 1=w414:i16)
        n256 = Negate(x=w414) -> (-x=w413:i16)
        n257 = Add(x=w412, y=w413) -> (x+y=w411:i16)
        n258 = call <vilib>:"NT Write Number.vi"("Numeric"=w411, "Name"=w410) -> ()  [unwired: 9 in, 1 out]
      }
      event "Test Ring": Value Change {
        # "When a test mode helper value is selected from the ring,\nset the tree item's variable to the string value"
        n259 = event-data() -> ("NewVal"=w420:u16)  [unwired: 1 in]
        n260 = property on="Test Ring" class="Ring (strict)"() -> ("Strings []"=w421:string[])  [unwired: 2 in, 2 out]
        n261 = Index Array(array=w421, index=w420) -> (element=w419:string)
        n262 = call <vilib>:"NT Write String.vi"("String"=w419, "Name"=w418) -> ()  [unwired: 9 in, 1 out]
      }
      event "Rec Mode": Value Change {
        # "Update globals for recording mode and path to read log from.\nClear when logging and let NetworkTables set path for vision to\nuse."
        n263 = event-data() -> ("NewVal"=w431:enum32{"Stop", "Record", "Playback"})  [unwired: 1 in]
        n264 = global write "WPI_DashboardLogging Global.vi" "Logging Filename"(path "") -> ()
        n265 = case shown="\"Playback\"" w431 {
          tunnel: w430 -> [_ w433 w441]
          tunnel: [_ _ w440] -> w427
          tunnel: [_ _ w439] -> _
          tunnel: w425 -> [_ _ w437]
          tunnel: cluster{i32, i32} {-250, 170} -> [_ _ w436]
          tunnel: [_ _ T21 {"Image Size"=TRUE, "Image Type"=TRUE, "Pixel Value"=TRUE, "ROI Information"=TRUE, "Zoom Factor"=FALSE} ("Image Information Shown:All Elements")] -> w423
          tunnel: [_ _ TRUE ("Zoom Factor")] -> w422
          frame Default {
          }
          frame "Stop", "Record" {
            # "Place Window too"
            n266 = invoke class="VI" method="FP.Close"(reference=w433) -> (reference out=w432:refnum<vi>)  [unwired: 2 in, 2 out]
            n267 = invoke class="VI" method="Abort VI"(reference=w432) -> ()  [unwired: 2 in, 3 out]
          }
          frame "Playback" {
            n268 = call "Open Playback Panel.vi"("Offset"=w436, "DB VI Ref"=w437, "Playback in"=w441) -> ("Playback out"=w438:refnum<vi>)  [unwired: 8 in]
            n269 = register-events(w438) -> (reference out=w440:refnum<event-registration>, error out=w439:errorcluster)  [unwired: 2 in]
          }
        }
        n270 = global write "WPI_DashboardLogging Global.vi" "Recording"(w431) -> ()
        n271 = property on="Camera Image" class="ImageControl"("Image Information Shown"=w423, "Image Information Visible"=w422) -> ()  [unwired: 2 in, 2 out]
        n272 = call <vilib>:"WPI_DashboardNT Log FieldName Cache.vi"("Operation"=enum16{"Lookup/Add", "Index", "Clear"}."Clear") -> ()  [unwired: 8 in, 3 out]
      }
      event Panel Close {
        w442 = enum32{"Stop", "Record", "Playback"}."Stop" ("Rec Mode")
        # "Playback window has been closed, abort"
        n273 = event-data() -> ()  [unwired: 1 in, 4 out]
        n274 = local write "Rec Mode"(w442) -> ()
        n275 = global write "WPI_DashboardLogging Global.vi" "Recording"(w442) -> ()
      }
      event Panel Close {
        # "Abort playback window and ourself"
        n276 = event-data() -> ()  [unwired: 1 in, 4 out]
        n277 = invoke class="VI" method="FP.Close"(reference=w447) -> (reference out=w446:refnum<vi>)  [unwired: 2 in, 2 out]
        n278 = invoke class="VI" method="Abort VI"(reference=w446) -> (error out=w445:errorcluster)  [unwired: 2 in, 2 out]
        n279 = invoke class="VI" method="Abort VI"(error in=w445) -> ()  [unwired: 2 in, 3 out]
      }
      event "Vision": Value Change {
        # "Enable/Disable Compression slider.\nHW USB is hard-coded into the camera"
        n280 = event-data() -> ("NewVal"=w453:u16)  [unwired: 1 in]
        n281 = Equal?(x=w453, y=u32 2 ("milliseconds to wait")) -> (x = y?=w451:bool)
        n282 = Select(t=T22."Disabled and Grayed Out" ("Disabled"), s=w451, f=T22."Enabled" ("Disabled")) -> (s? t:f=w448:T22)
        n283 = property on="Compression" class="Slide (strict)"("DisabledEnum"=w448) -> ()  [unwired: 2 in, 2 out]
      }
    }
  }
  n284 = while {
    tunnel: w42 -> [w456]
    i -> [w459]
    stop <- FALSE stop-if-true
    n285 = Wait (ms)(milliseconds to wait=u32 100) -> ()  [unwired: 1 out]
    n286 = case shown="\"Playback\"" "Rec Mode" {
      tunnel: w459 -> [_ _ w474]
      tunnel: [u32 2829099 ("Base Color") u32 11141120 ("Target Color") w463] -> w455
      frame "Stop", Default {
        # "Reset the color, extra updates don't cost much"
      }
      frame "Record" {
      }
      frame "Playback" {
        # "Playback"
        n287 = Quotient & Remainder(x=w474, y=u32 50 ("milliseconds to wait")) -> (x-y*floor(x/y)=w470:u32)  [unwired: 1 out]
        n288 = Divide(x=w470, y=u32 50 ("milliseconds to wait")) -> (x/y=w467:dbl)
        n289 = Multiply(x=6.283185307179586, y=w467) -> (x*y=w472:dbl)
        n290 = Sine(x=w472) -> (sin(x)=w471:dbl)
        n291 = Absolute Value(x=w471) -> (abs(x)=w464:dbl)
        n292 = call "Interpolate RGB Color.vi"("Proportion"=w464, "Target Color"=u32 30976, "Base Color"=u32 2829099) -> ("Result Color"=w463:u32)  [unwired: 8 in]
      }
    }
    n293 = property class="Pane"(reference=w456, "PaneColor"=w455) -> ()  [unwired: 1 in, 2 out]
  }
  n294 = property on="On/Off" class="Bool (strict)"("Visible"=w15) -> ()  [unwired: 2 in, 2 out]
  n295 = property on="Motor" class="Clust (strict)"("Visible"=w15) -> ()  [unwired: 2 in, 2 out]
  n296 = property on="Progress" class="Clust (strict)"("Visible"=w15) -> ()  [unwired: 2 in, 2 out]
  n297 = property on="Test Ring" class="Ring (strict)"("Visible"=w15) -> ()  [unwired: 2 in, 2 out]
  n298 = property on="Rev/Fwd" class="Clust (strict)"("Visible"=w15) -> ()  [unwired: 2 in, 2 out]
  n299 = while {
    tunnel: u16 1741 ("timeout ms (25000)") -> [w478]
    stop <- FALSE stop-if-true
    n300 = TCP Create Listener(10:w478) -> (0:w476:errorcluster, 3:w477:refnum<k5>)  [unwired: 4 in, 1 out]
    n301 = case shown="No Error" w476 {
      selector: w476 -> [w479 _]
      tunnel: w477 -> [w480 _]
      frame No Error {
        n302 = while {
          tunnel: w480 -> [w485]
          tunnel: w479 -> [w483]
          stop <- FALSE stop-if-true
          n303 = TCP Wait On Listener(8:w483, 11:w485) -> (0:w482:errorcluster, 4:w484:refnum<k5>)  [unwired: 2 in, 3 out]
          n304 = case shown="Error" w482 {
            frame No Error {
            }
            frame Error {
              n305 = Wait (ms)(milliseconds to wait=u32 100) -> ()  [unwired: 1 out]
            }
          }
          n306 = local write "TCP"(w484) -> ()
        }
      }
      frame Error {
      }
    }
  }
  n307 = property on="Camera Settings" class="Clust (strict)"("Visible"=w15) -> ()  [unwired: 2 in, 2 out]
  n308 = local write "DB Camera Config"(w15) -> ()
  n309 = global write "WPI_DashboardLogging Global.vi" "Recording"(w36) -> ()
  n310 = local write "Rec Mode"(w36) -> ()
